vi "ConvertArrayToCSVString.vi"(11 "Array":dbl[](array[numeric])) -> (3 "CSV String":string)   [LabVIEW 2012, in "LV-Utilities.lvlib"]
uses:
  LV-Utilities.lvlib
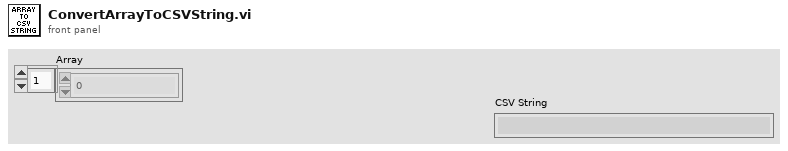
[diagram p1: front panel]
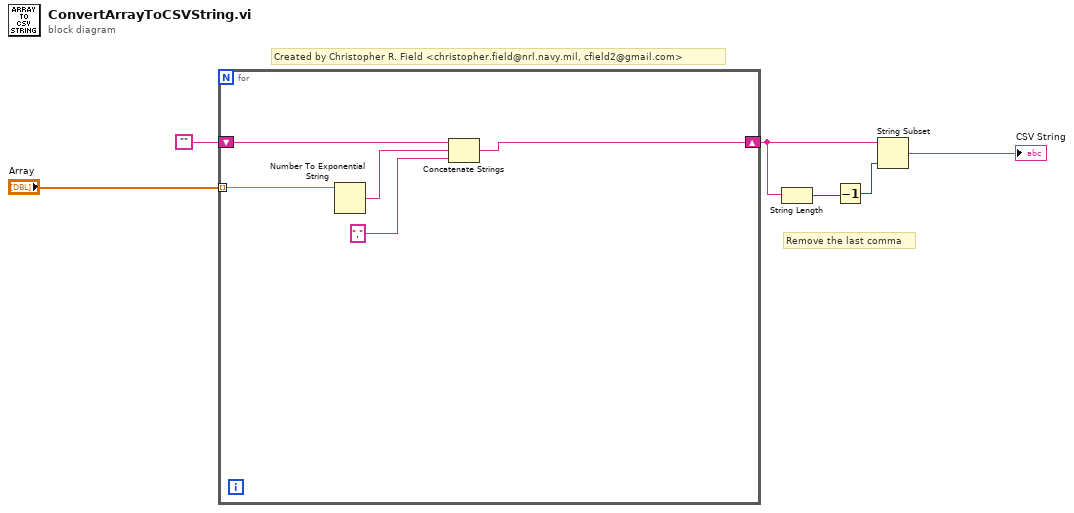
[diagram p0: block diagram]
diagram:
  # "Created by Christopher R. Field <christopher.field@nrl.navy.mil, cfield2@gmail.com>"
  # "Remove the last comma"
  n1 = for {
    tunnel: "Array" -> [w11] mode=indexing
    shift-right: [w8] -> w4
    shift-left: "" -> [w10]
    n2 = Number To Exponential String(number=w11) -> (E-format string=w9:string)  [unwired: 3 in]
    n3 = Concatenate Strings(w10, w9, ",") -> (w8:string)
  }
  n4 = String Length(string=w4) -> (length=w3:i32)
  n5 = Decrement(x=w3) -> (x-1=w2:i32)
  n6 = String Subset(string=w4, length (rest)=w2) -> (substring=→"CSV String":string)  [unwired: 1 in]
